vi "Set Sensor Mov wrapper.vi"(7 "pSensorMovObj":T1, 8 "error in (no error)":errorcluster caption="错误输入（无错误）", 9 "iSensor":u16(ring) items=["S1 rising"=2, "S1 falling"=3, "S2 rising"=4, "S2 falling"=5, "S3 rising"=6, "S3 falling"=7], 10 "dwCanNodeId":u32, 11 "dwDevIndex":u32) -> (0 "error out":errorcluster caption="错误输出", 3 "function return":u32)   [LabVIEW 2016, in "UISimCanFunc_wrapper.lvlib"]
doc: "_declspec (dllexport) DWORD SetSensorMov_wrapper(DWORD dwDevIndex, DWORD dwCanNodeId, INT iSensor, P_SENSOR_MOVE_PARA_OBJ pSensorMovObj);"
uses:
  <userlib>/UISimCanFunc_wrapper/UISimCanFunc_wrapper.lvlib
  <userlib>/UISimCanFunc_wrapper/UISimCanFunc_wrapper.dll
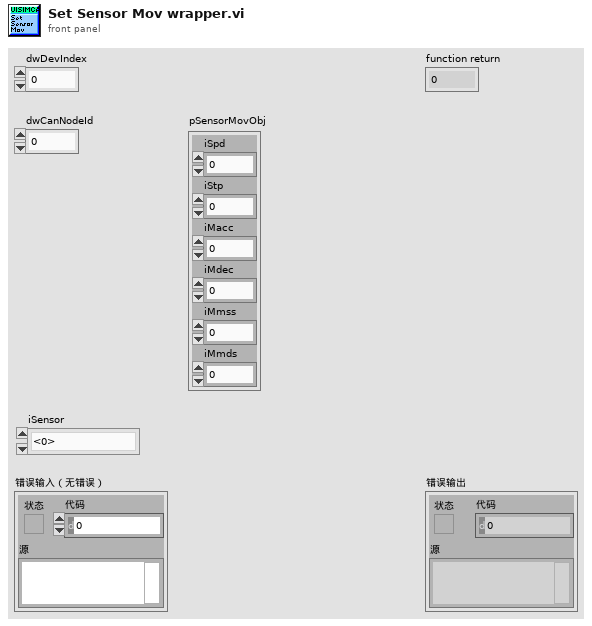
[diagram p1: front panel]
types:
  T1 = cluster{"iSpd":i32, "iStp":i32, "iMacc":i32, "iMdec":i32, "iMmss":i32, "iMmds":i32}
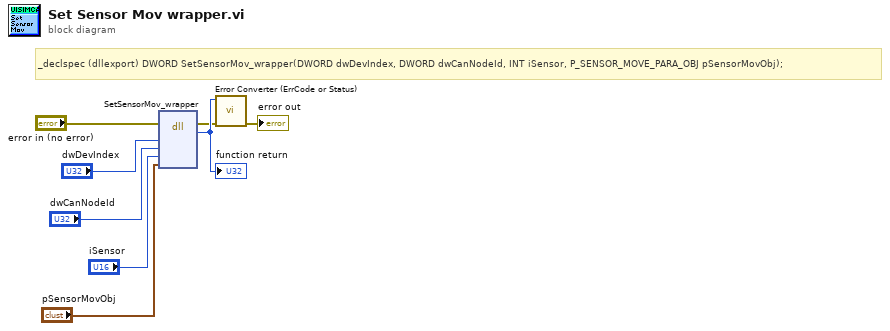
[diagram p0: block diagram]
diagram:
  # "_declspec (dllexport) DWORD SetSensorMov_wrapper(DWORD dwDevIndex, DWORD dwCanNodeId, INT iSensor, P_SENSOR_MOVE_PARA_OBJ pSensorMovObj);"
  n1 = dll-call lib="C:/Program Files (x86)/National Instruments/LabVIEW 2016/user.lib/UISimCanFunc_wrapper/UISimCanFunc_wrapper.*" fn="SetSensorMov_wrapper"(error in="error in (no error)", "dwDevIndex"="dwDevIndex", "dwCanNodeId"="dwCanNodeId", "iSensor"="iSensor", "pSensorMovObj"="pSensorMovObj") -> (error out=w2:errorcluster, w8:u32)  [unwired: 6 in, 1 out]
  "function return" <- w8
  n2 = call <userlib>:"Error Converter (ErrCode or Status).vi"("error in (no error)"=w2, "error code"=w8) -> ("error out"=→"error out":errorcluster)  [unwired: 9 in]
